vi "H5PTget_num_packets.vi"(3 "table_id":i32, 9 "error in (no error)":errorcluster) -> (0 "status":i32, 2 "nrecords":i64, 6 "error out":errorcluster)   [LabVIEW 2009]
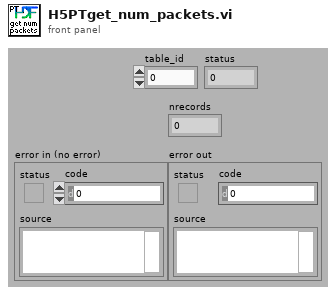
[diagram p1: front panel]
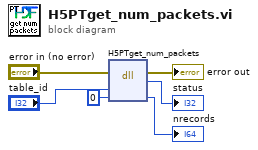
[diagram p0: block diagram]
diagram:
  n1 = dll-call lib="hdf5_hldll" fn="H5PTget_num_packets"(error in="error in (no error)", "table_id"="table_id", "nrecords"=i64 0) -> (error out=→"error out":errorcluster, "return type"=→"status":i32, "nrecords"=→"nrecords":i64)  [unwired: 3 in, 1 out]
